vi "Freeze PID.vi"(0 "Run Profile":bool, 5 "Controller CMDs":dbl[](array[numeric]), 7 "Controller Config":T1, 9 "Power Relay":T3) -> ()   [LabVIEW 2019]
uses:
  Controls/Controller Config.ctl
  Type Defs/Controller Names.ctl
  Controls/Power Supply Global Mode.ctl
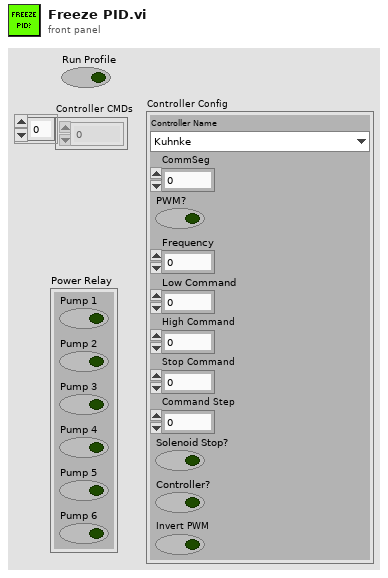
[diagram p1: front panel]
types:
  T1 = typedef "Controller Config.ctl" = cluster{"Controller Name":T2, "CommSeg":i32, "PWM?":bool, "Frequency":i32, "Low Command":dbl, "High Command":dbl, "Stop Command":dbl, "Command Step":dbl, "Solenoid Stop?":bool, "Controller?":bool, "Invert PWM":bool}
  T2 = typedef "Controller Names.ctl" = enum16{"Kuhnke", "Helbako BLDC", "Conti", "Hella BLDC OL PWM", "Hella BLDC Turbine OL PWM", "Hella BLDC Pressure", "Helbako (old)", "TI PWM", "PSA", "Hella Gas", "Hella Diesel", "8 Comm", "10 Comm", "8 Comm Hella", "10 Comm Hella", "8 Comm Omron", "10 Comm Omron", "8 Comm Nissan", "10 Comm Nissan", "8 Comm Hella (for FCA)", "Mazda BLDC"}
  T3 = cluster{"Pump 1":bool, "Pump 2":bool, "Pump 3":bool, "Pump 4":bool, "Pump 5":bool, "Pump 6":bool}
  T4 = typedef "Power Supply Global Mode.ctl" = enum16{"Write Setpoint", "Write FreezePID", "Read"}
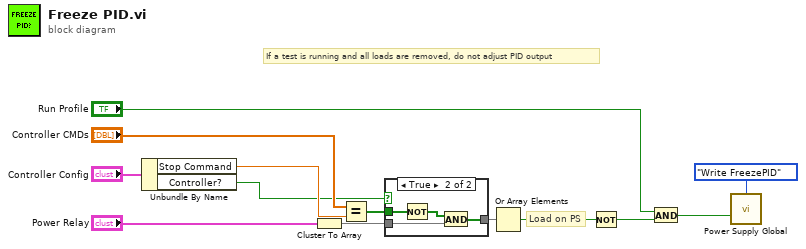
[diagram p0: block diagram]
diagram:
  # "If a test is running and all loads are removed, do not adjust PID output"
  # "Load on PS"
  n1 = Unbundle By Name("Controller Config") -> ("Stop Command"=w4:dbl, "Controller?"=w3:bool)
  n2 = Cluster To Array(cluster="Power Relay") -> (array=w7:bool[])
  n3 = Equal?(x="Controller CMDs", y=w4) -> (x = y?=w13:bool[])
  n4 = case shown="True" w3 {
    tunnel: w13 -> [_ w18]
    tunnel: w7 -> [w14 w16]
    tunnel: [w14 w15] -> w8
    frame False {
    }
    frame True {
      n5 = Not(x=w18) -> (.not. x?=w17:bool[])
      n6 = And(x=w17, y=w16) -> (x .and. y?=w15:bool[])
    }
  }
  n7 = Or Array Elements(Boolean array=w8) -> (logical OR=w9:bool)
  n8 = Not(x=w9) -> (.not. x?=w10:bool)
  n9 = And(x="Run Profile", y=w10) -> (x .and. y?=w1:bool)
  n10 = call "Power Supply Global.vi"("PS Global Mode"=Power_Supply_Global_Mode."Write FreezePID", "FreezePID"=w1) -> ()  [unwired: 9 in, 5 out]
